vi "Pre-Install Custom Action.vi"(10 "Variant":variant) -> (0 "error out":errorcluster)   [LabVIEW 2013]
uses:
  <vilib>/nisyscfg/Get Installed Components.vi
  <vilib>/nisyscfg/nisyscfg.lvlib
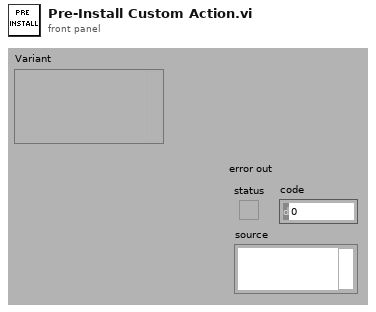
[diagram p1: front panel]
types:
  T1 = typedef "nisyscfg.lvlib/Software 1.2.ctl" = cluster{"title":string, "description":string, "ID":string, "version":string, "component type":T2}
  T2 = typedef "nisyscfg.lvlib/Component Type.ctl" = u32
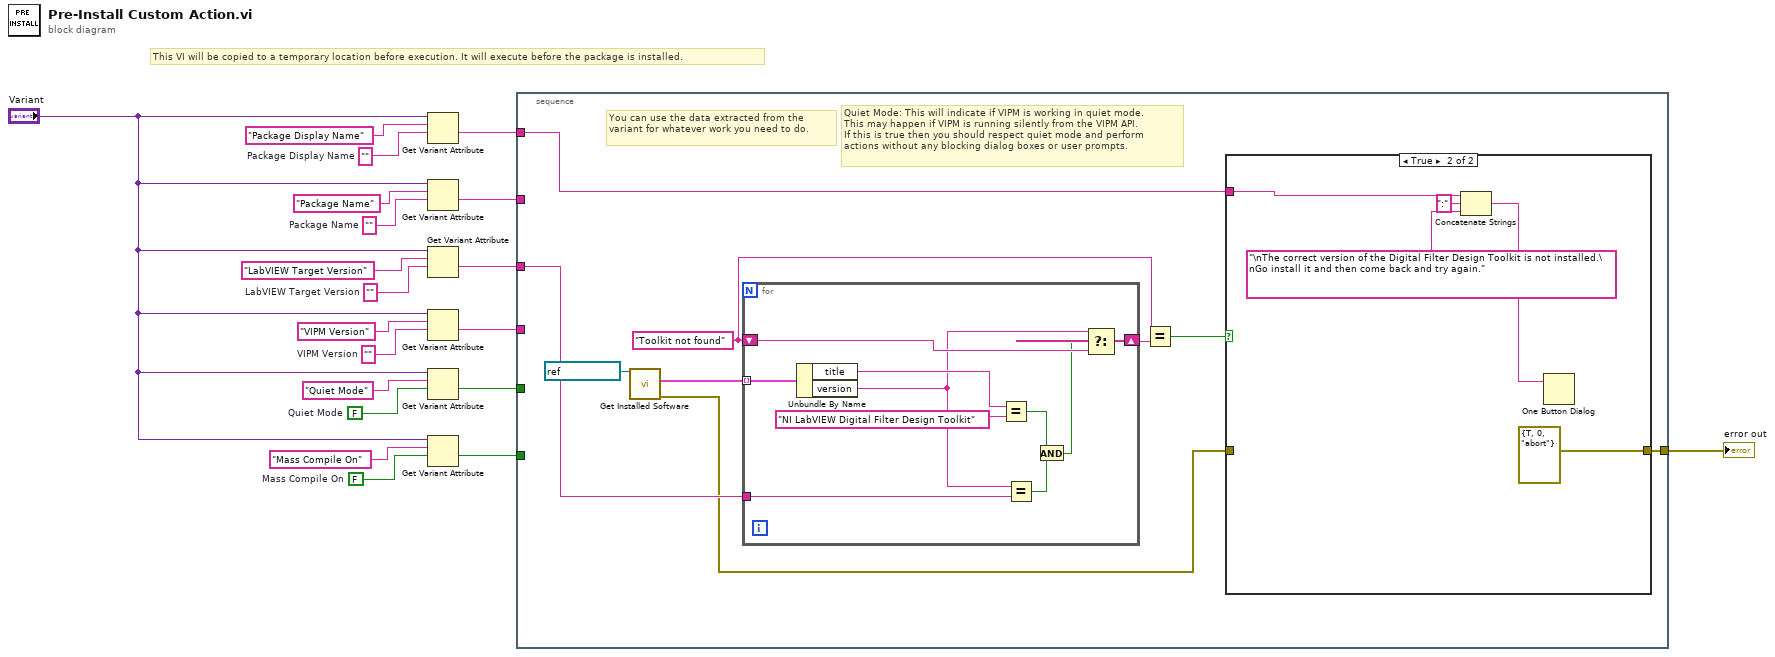
[diagram p0: block diagram]
diagram:
  w2 = FALSE  # Mass Compile On
  w4 = ""  # Package Display Name
  w11 = FALSE  # Quiet Mode
  w14 = ""  # VIPM Version
  w16 = ""  # LabVIEW Target Version
  w18 = ""  # Package Name
  # "This VI will be copied to a temporary location before execution. It will execute before the package is installed."
  n1 = Get Variant Attribute(Variant="Variant", name="Package Display Name", default value (empty Variant)=w4) -> (value=w10:string)  [unwired: 1 in, 3 out]
  n2 = Get Variant Attribute(Variant="Variant", name="Package Name", default value (empty Variant)=w18) -> (value=w9:string)  [unwired: 1 in, 3 out]
  n3 = Get Variant Attribute(Variant="Variant", name="LabVIEW Target Version", default value (empty Variant)=w16) -> (value=w8:string)  [unwired: 1 in, 3 out]
  n4 = Get Variant Attribute(Variant="Variant", name="VIPM Version", default value (empty Variant)=w14) -> (value=w7:string)  [unwired: 1 in, 3 out]
  n5 = Get Variant Attribute(Variant="Variant", name="Quiet Mode", default value (empty Variant)=w11) -> (value=w6:bool)  [unwired: 1 in, 3 out]
  n6 = Get Variant Attribute(Variant="Variant", name="Mass Compile On", default value (empty Variant)=w2) -> (value=w5:bool)  [unwired: 1 in, 3 out]
  n7 = stacked-sequence {
    tunnel: w10 -> [w21]
    tunnel: w9 -> [_]
    tunnel: w8 -> [w26]
    tunnel: w7 -> [_]
    tunnel: w6 -> [_]
    tunnel: w5 -> [_]
    tunnel: [w23] -> w1
    frame #0 {
      w24 = "Toolkit not found" ("version")
      # "Quiet Mode: This will indicate if VIPM is working in quiet mode.\nThis may happen if VIPM is running silently from the VIPM API.\nIf this is true then you should respect quiet mode and perform\nactions without any blocking dialog boxes or user prompts."
      # "You can use the data extracted from the variant for whatever work you need to do."
      n8 = call-poly <vilib>:"Get Installed Software.vi"("Session in"=refnum<k21> "localhost") -> ("error out"=w22:errorcluster, "Software Components"=w28:T1[])  [unwired: 8 in, 1 out]
      n9 = for {
        tunnel: w28 -> [w45] mode=indexing
        shift-right: [w42] -> w29
        shift-left: w24 -> [w41]
        tunnel: w26 -> [w36]
        n10 = Unbundle By Name(w45) -> ("title"=w43:string, "version"=w40:string)
        n11 = Equal?(x=w43, y="NI LabVIEW Digital Filter Design Toolkit" ("regular expression")) -> (x = y?=w39:bool)
        n12 = Equal?(x=w40, y=w36) -> (x = y?=w38:bool)
        n13 = And(x=w39, y=w38) -> (x .and. y?=w37:bool)
        n14 = Select(t=w40, s=w37, f=w41) -> (s? t:f=w42:string)
      }
      n15 = Equal?(x=w24, y=w29) -> (x = y?=w25:bool)
      n16 = case shown="True" w25 {
        tunnel: [w30 errorcluster {"status"=TRUE, "code"=0, "source"="abort"} ("error out")] -> w23
        tunnel: w22 -> [w30 _]
        tunnel: w21 -> [_ w33]
        frame False {
        }
        frame True {
          n17 = Concatenate Strings(w33, ":" ("string"), "\nThe correct version of the Digital Filter Design Toolkit is not installed.\nGo install it and then come back and try again." ("message")) -> (w31:string)
          n18 = One Button Dialog(message=w31) -> ()  [unwired: 1 in, 1 out]
        }
      }
    }
  }
  "error out" <- w1
